vi "Read Multiple Channels with Simple Header.vi"() -> ()   [LabVIEW 2012]
uses:
  <vilib>/Utility/file.llb/Read From Spreadsheet File (string).vi
panel:
  out "所有通道":dbl[][](graph)
  out "二维字符串数组":string[][](array[string])
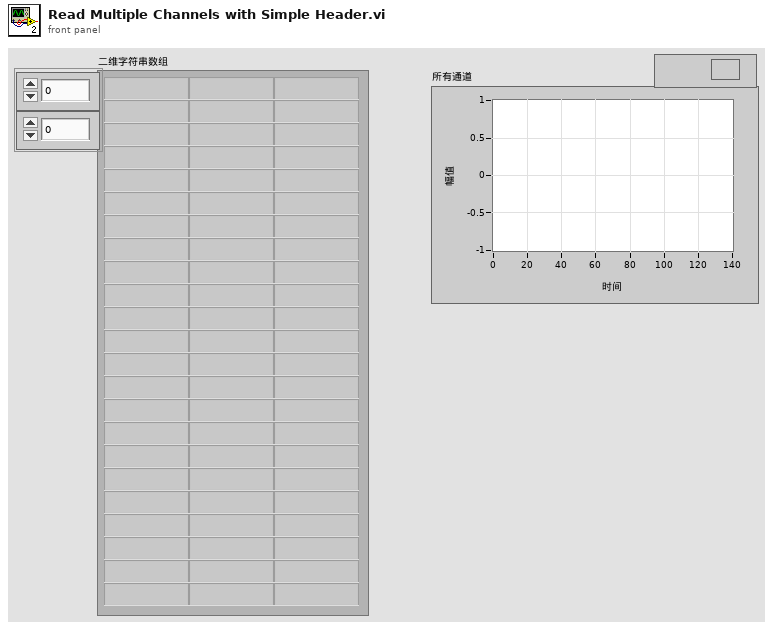
[diagram p1: front panel]
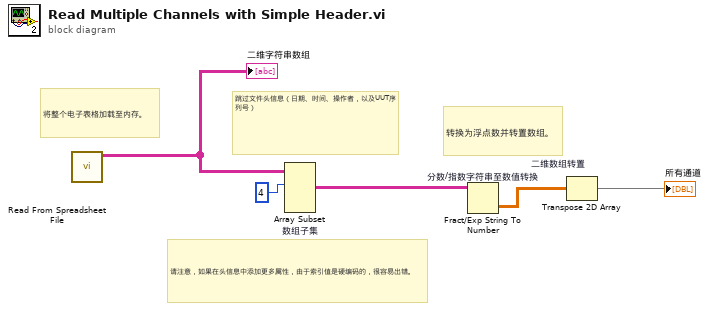
[diagram p0: block diagram]
diagram:
  # "请注意，如果在头信息中添加更多属性，由于索引值是硬编码的，很容易出错。"
  # "转换为浮点数并转置数组。"
  # "跳过文件头信息（日期、时间、操作者，以及UUT序列号）"
  # "将整个电子表格加载至内存。"
  n1 = call-poly <vilib>:"Read From Spreadsheet File.vi"() -> ("all rows"=w1:string[][])  [unwired: 7 in, 4 out]
  "二维字符串数组" <- w1
  n2 = Array Subset "数组子集"(array=w1, index (row)=4 ("索引")) -> (w3:string[][])  [unwired: 3 in]
  n3 = Fract/Exp String To Number "分数/指数字符串至数值转换"(string=w3) -> (number=w5:dbl[][])  [unwired: 3 in, 1 out]
  n4 = Transpose 2D Array "二维数组转置"(2D array=w5) -> (transposed array=→"所有通道":dbl[][])
